vi "VoltageScan_Probecard.vi"() -> ()   [LabVIEW 2016]
uses:
  <vilib>/Utility/file.llb/Read Delimited Spreadsheet (DBL).vi
  <instrlib>/Keithley 24XX/Public/Data/Read (Single Point).vi
  <vilib>/Utility/file.llb/Write Delimited Spreadsheet (string).vi
  <instrlib>/Keithley 24XX/Keithley 24XX.lvlib
  <instrlib>/Agilent 428X Series/Agilent 428X Series.lvlib
panel:
  in  "Stop":bool
  in  "Sensor type":enum16{"6''", "8''", "One channel"}(ring)
  out "Channels":cluster{i32[], dbl[]}[](graph) caption="XY Graph"
  in  "Voltage Delay (s)":dbl=0.5 format="%#_13g"
  out "Secondary Value":dbl format="%^.4e"
  out "Primary Value":dbl format="%^.4e"
  out "Data Status":bool=TRUE
  in  "VISA resource name LCR":refnum<visa-resource-name>
  in  "Short (F:OFF)":bool
  in  "Open (F:OFF)":bool
  in  "Imp Type (0: CPD)":u32(ring) items=["CPD", "CPQ", "CPG", "CPRP", "CSD", "CSQ", "CSRS", "LPQ", "LPD", "LPG", "LPRP", "LSD", "LSQ", "LSRS", "RX", "ZTD", "ZTR", "GB", "YTD", "YTR"]
  in  "Freq Value (Hz)(1.0 kHz)":dbl=1000.0 min=20.0 max=30000000.0 step=10.0 format="%.4e"
  in  "Voltage Level (V)(1.0V)":dbl=1.0 min=0.0 max=20.0 step=0.1 format="%.4f"
  in  "Compliance  Level (uA)":dbl=0.1
  in  "Enable Voltage Auto Range (T:Enable)":bool=TRUE
  in  "Voltage Manual Range (1.0)":dbl=1.0
  in  "Serial Configuration":T1={"Baud Rate"=9600, "Parity"=0, "Data Bits"=8, "Stop Bits"=10, "Flow Control"=0} {"Flow Control" items=["None", "XON/XOFF", "RTS/CTS", "XON/XOFF & RTS/CTS", "DTR/DSR", "XON/XOFF & DTR/DSR"]; "Stop Bits" items=["1.0"=10, "1.5"=15, "2.0"=20]; "Data Bits" items=["7"=7, "8"=8]; "Parity" items=["None", "Odd", "Even", "Mark", "Space"]; "Baud Rate" items=["300"=300, "600"=600, "1200"=1200, "2400"=2400, "4800"=4800, "9600"=9600, "19200"=19200]}
  in  "VISA resource name":refnum<visa-resource-name>
  out "error out":errorcluster
  in  "Open after execution?":bool
  out "Output file":path
  in  "Output file":string="test.txt"
  out "Current voltage [V]":dbl
  out "Current channel":i32
  in  "Switch Delay (s)":dbl=0.01 format="%#_13g"
  out "Voltages":cluster{"X":dbl[], "Y":dbl[]}[](graph) caption="XY Graph"
  out "Input file":path
  in  "Measurement type":enum16{"IV", "CV", "Test"}(ring)=enum."Test"
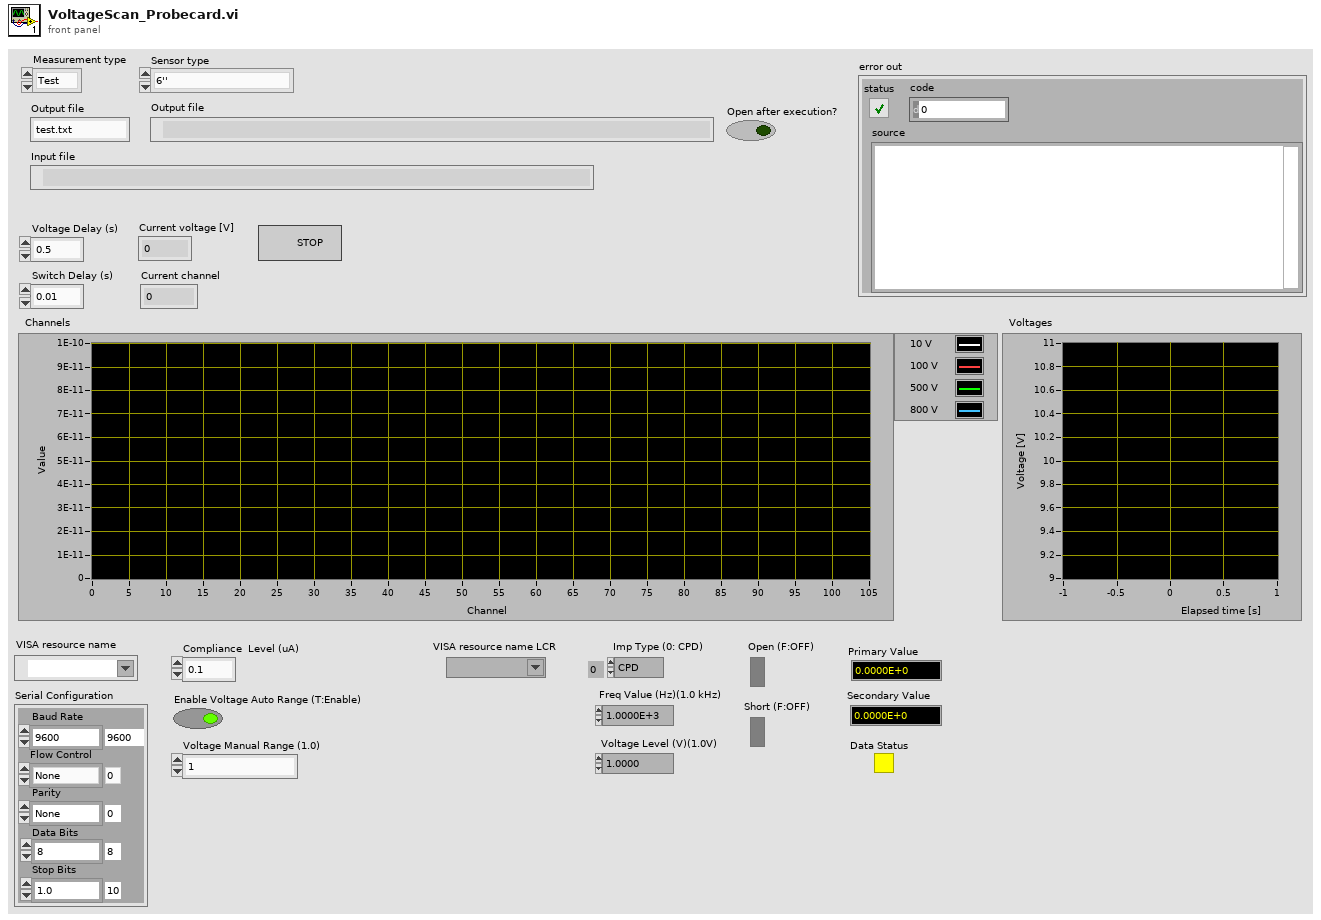
[diagram p1: front panel]
types:
  T1 = cluster{"Baud Rate":u32, "Parity":u16, "Data Bits":u16, "Stop Bits":u16, "Flow Control":u16}
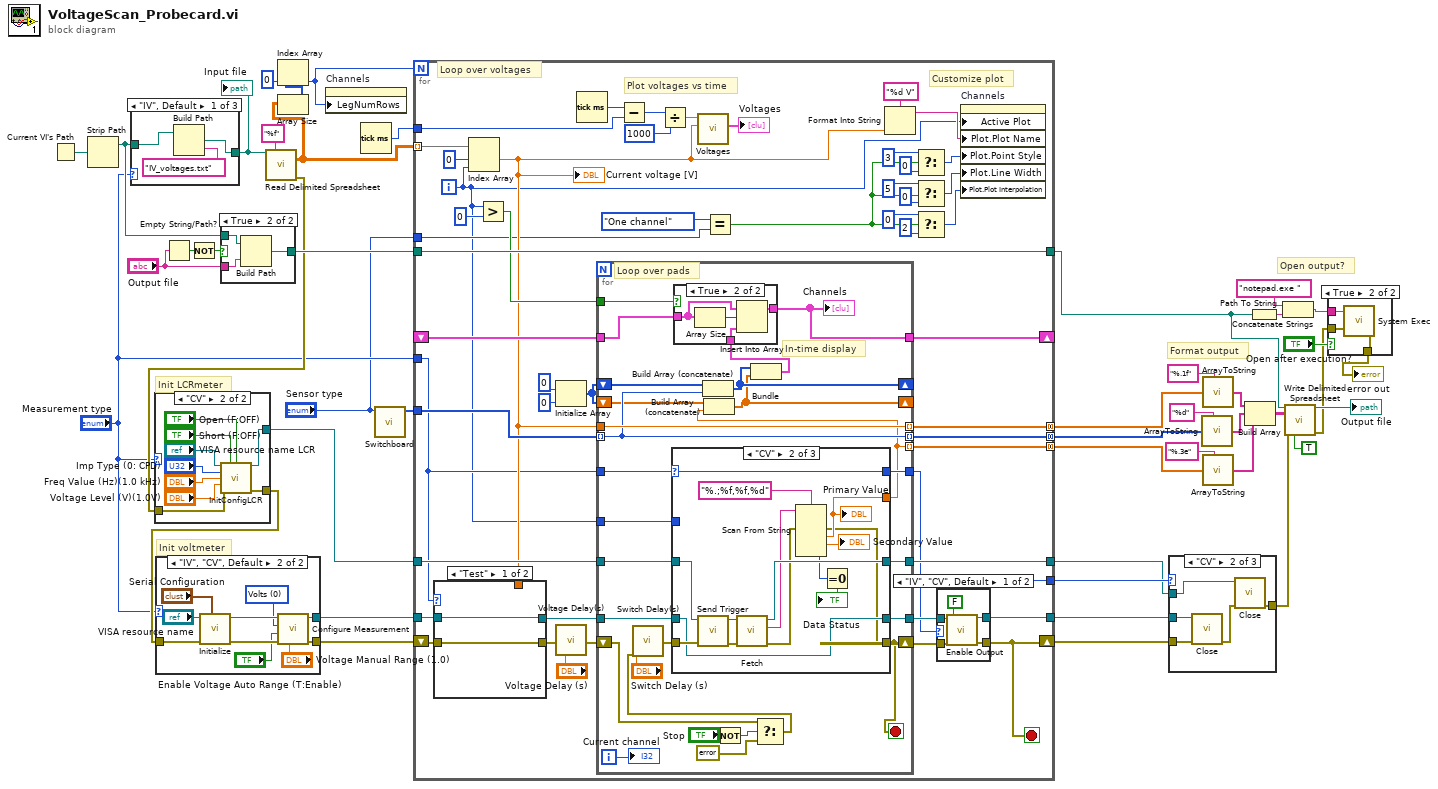
[diagram p0: block diagram]
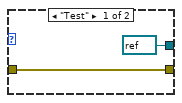
[diagram p2: hidden frame]
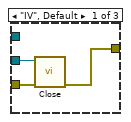
[diagram p3: hidden frame]
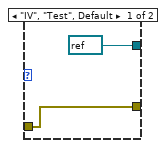
[diagram p5: hidden frame]
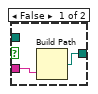
[diagram p7: hidden frame]
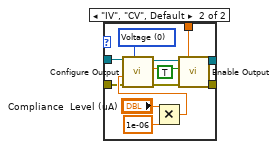
[diagram p9: hidden frame]
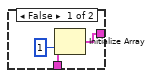
[diagram p10: hidden frame]
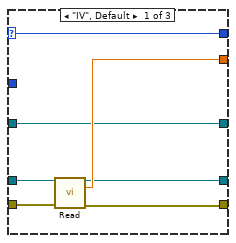
[diagram p11: hidden frame]
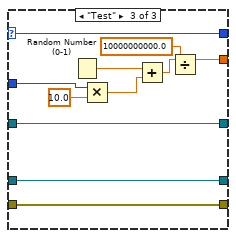
[diagram p12: hidden frame]
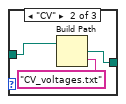
[diagram p13: hidden frame]
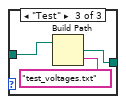
[diagram p14: hidden frame]
diagram:
  # "Init LCRmeter"
  # "Init voltmeter"
  # "Format output"
  # "Open output?"
  n1 = Current VI's Path() -> (path=w44:path)
  n2 = Strip Path(path=w44) -> (stripped path=w38:path)  [unwired: 1 out]
  n3 = case shown="\"IV\", Default" "Measurement type" {
    tunnel: [w46 w49 w52] -> w19
    tunnel: w38 -> [w48 w50 w53]
    frame "IV", Default {
      n4 = Build Path(base path=w48, name or relative path="IV_voltages.txt") -> (appended path=w46:path)
    }
    frame "CV" {
      n5 = Build Path(base path=w50, name or relative path="CV_voltages.txt") -> (appended path=w49:path)
    }
    frame "Test" {
      n6 = Build Path(base path=w53, name or relative path="test_voltages.txt") -> (appended path=w52:path)
    }
  }
  "Input file" <- w19
  n7 = Empty String/Path?(string/path="Output file") -> (empty?=w36:bool)
  n8 = Not(x=w36) -> (.not. x?=w34:bool)
  n9 = case shown="True" w34 {
    tunnel: "Output file" -> [w56 w59]
    tunnel: w38 -> [_ w58]
    tunnel: [w55 w57] -> w16
    frame False {
      n10 = Build Path(name or relative path=w56) -> (appended path=w55:path)  [unwired: 1 in]
    }
    frame True {
      n11 = Build Path(base path=w58, name or relative path=w59) -> (appended path=w57:path)
    }
  }
  n12 = call-poly <vilib>:"Read Delimited Spreadsheet.vi"("file path (dialog if empty)"=w19, "format (%.3f)"="%f") -> ("all rows"=w41:dbl[][], "error out"=w12:errorcluster)  [unwired: 8 in, 4 out]
  n13 = case shown="\"CV\"" "Measurement type" {
    tunnel: w12 -> [w61 w64]
    tunnel: [w61 w63] -> w11
    tunnel: [refnum<visa-resource-name> refnum ("VISA resource name out") w62] -> w10
    frame "IV", "Test", Default {
    }
    frame "CV" {
      n14 = call "InitConfigLCR.vi"("VISA resource name LCR"="VISA resource name LCR", "Short (F:OFF)"="Short (F:OFF)", "Open (F:OFF)"="Open (F:OFF)", "Imp Type (0: CPD)"="Imp Type (0: CPD)", "Freq Value (Hz)(1.0 kHz)"="Freq Value (Hz)(1.0 kHz)", "Voltage Level (V)(1.0V)"="Voltage Level (V)(1.0V)", "error in (no error)"=w64) -> ("VISA resource name out"=w62:refnum<visa-resource-name>, "error out"=w63:errorcluster)  [unwired: 7 in]
    }
  }
  n15 = case shown="\"IV\", \"CV\", Default" "Measurement type" {
    tunnel: [refnum<visa-resource-name> refnum ("VISA resource name out") w76] -> w15
    tunnel: [w72 w75] -> w14
    tunnel: w11 -> [w72 w74]
    frame "Test" {
    }
    frame "IV", "CV", Default {
      w79 = u16 0 items=["Volts", "Current", "Resistance"] ("Function (0: Volts)")
      n16 = call <instrlib>:"Initialize.vi"("Serial Configuration"="Serial Configuration", "error in (no error)"=w74, "VISA resource name"="VISA resource name") -> ("error out"=w80:errorcluster, "VISA resource name out"=w81:refnum<visa-resource-name>)  [unwired: 7 in]
      n17 = call <instrlib>:"Configure Measurement.vi"("Manual Range (1.0)"="Voltage Manual Range (1.0)", "error in (no error)"=w80, "Enable Auto Range (T:Enable)"="Enable Voltage Auto Range (T:Enable)", "Function (0: Volts)"=w79, "VISA resource name"=w81) -> ("error out"=w75:errorcluster, "VISA resource name out"=w76:refnum<visa-resource-name>)  [unwired: 5 in]
    }
  }
  n18 = Array Size(array=w41) -> (size(s)=w43:i32[])
  n19 = Index Array(array=w43, index=0) -> (element=w2:i32)
  n20 = property on="Channels" class="XYGraph (strict)"("LegNumRows"=w2) -> ()  [unwired: 2 in, 2 out]
  n21 = Tick Count (ms)() -> (millisecond timer value=w4:u32)
  n22 = call "Switchboard.vi"("Sensor type"="Sensor type") -> ("Output config"=w40:i32[])  [unwired: 10 in]
  n23 = for {
    N: w2 -> [_]
    tunnel: w41 -> [w132] mode=indexing
    tunnel: w40 -> [w129]
    tunnel: [w127] -> w26 mode=concatenating
    tunnel: [w125] -> w24 mode=concatenating
    tunnel: [w126] -> w25 mode=concatenating
    tunnel: w16 -> [w124]
    tunnel: [w124] -> w13
    tunnel: w15 -> [w123]
    tunnel: [w122] -> w5
    tunnel: "Measurement type" -> [w96]
    shift-right: [w100] -> w3
    shift-left: w14 -> [w117]
    tunnel: w10 -> [w116]
    tunnel: [w112] -> w9
    tunnel: [w118] -> w8
    shift-right: [w110] -> _
    shift-left: _ -> [w109]
    tunnel: w4 -> [w103]
    tunnel: "Sensor type" -> [w94]
    i -> [w83]
    stop <- w100 stop-if-true
    # "Plot voltages vs time"
    # "Customize plot"
    # "Loop over voltages"
    n24 = Index Array(array=w132, index #1=0 ("index"), index #2=w83) -> (element #1=w97:dbl)  [unwired: 1 out]
    "Current voltage [V]" <- w97
    n25 = case shown="\"Test\"" w96 {
      tunnel: w123 -> [w141 w146]
      tunnel: w97 -> [_ w145]
      tunnel: [w141 w144] -> w121
      tunnel: w117 -> [w140 w143]
      tunnel: [w140 w142] -> w114
      frame "Test" {
      }
      frame "IV", "CV", Default {
        w150 = u16 0 items=["Voltage", "Current"] ("Source Mode  (0: Voltage)")
        n26 = Multiply(x="Compliance  Level (uA)", y=1e-06) -> (x*y=w147:dbl)
        n27 = call <instrlib>:"Configure Output.vi"("Source Mode  (0: Voltage)"=w150, "error in (no error)"=w143, "Compliance  Level (0.1)"=w147, "Output Level (0)"=w145, "VISA resource name"=w146) -> ("error out"=w152:errorcluster, "VISA resource name out"=w153:refnum<visa-resource-name>)  [unwired: 5 in]
        n28 = call <instrlib>:"Enable Output.vi"("error in (no error)"=w152, "Enable Output (T: Enable)"=TRUE ("Enable Output"), "VISA resource name"=w153) -> ("error out"=w142:errorcluster, "VISA resource name out"=w144:refnum<visa-resource-name>)  [unwired: 7 in]
      }
    }
    n29 = Greater?(x=w83, y=0) -> (0:w111:bool)
    n30 = Initialize Array(0 ("dimension size"), 0 ("dimension size")) -> (w106:i32[])
    n31 = call "Voltage Delay(s)"("error in (no error)"=w114, "Delay Time (s)"="Voltage Delay (s)") -> ("error out"=w113:errorcluster)  [unwired: 9 in]
    n32 = Tick Count (ms)() -> (millisecond timer value=w105:u32)
    n33 = for {
      tunnel: w129 -> [w172] mode=indexing
      tunnel: [w172] -> w126 mode=indexing
      tunnel: [w170] -> w125 mode=indexing
      tunnel: w97 -> [w180]
      tunnel: [w180] -> w127 mode=indexing
      tunnel: w121 -> [w178]
      tunnel: [w177] -> w119
      tunnel: w96 -> [w179]
      shift-right: [w154] -> w120
      shift-left: w113 -> [w157]
      tunnel: w116 -> [w176]
      tunnel: [w175] -> w112
      tunnel: [w174] -> w118
      shift-right: [w168] -> _
      shift-left: w106 -> [w171]
      shift-right: [w167] -> _
      shift-left: w106 -> [w169]
      tunnel: w111 -> [w165]
      tunnel: w83 -> [w166]
      tunnel: w109 -> [w164]
      tunnel: [w162] -> w110
      i -> [w163]
      stop <- w154 stop-if-true
      # "In-time display"
      # "Loop over pads"
      n34 = Build Array (concatenate)(w171, w172) -> (w168:i32[])
      n35 = Not(x="Stop") -> (.not. x?=w158:bool)
      n36 = Select(t=w157, s=w158, f=errorcluster {"status"=TRUE, "code"=1, "source"="User stop"} ("User stop error")) -> (s? t:f=w155:errorcluster)
      n37 = call "Switch Delay(s)"("error in (no error)"=w155, "Delay Time (s)"="Switch Delay (s)") -> ("error out"=w156:errorcluster)  [unwired: 9 in]
      n38 = case shown="\"CV\"" w179 {
        selector: w179 -> [w189 w206 w220]
        tunnel: [w194 w198 w211] -> w170
        tunnel: w178 -> [w192 w197 w218]
        tunnel: w156 -> [w193 w204 w217]
        tunnel: [w191 w197 w218] -> w177
        tunnel: [w190 w195 w217] -> w154
        tunnel: w176 -> [w188 w207 w219]
        tunnel: [w189 w206 w220] -> w175
        tunnel: [w188 w205 w219] -> w174
        tunnel: w166 -> [_ _ w212]
        frame "IV", Default {
          n39 = call-poly <instrlib>:"Read.vi"("VISA resource name"=w192, "error in (no error)"=w193) -> ("VISA resource name out"=w191:refnum<visa-resource-name>, "Current"=w194:sgl, "error out"=w190:errorcluster)  [unwired: 7 in, 4 out]
        }
        frame "CV" {
          n40 = call <instrlib>:"Send Trigger.vi"("error in (no error)"=w204, "VISA resource name"=w207) -> ("error out"=w208:errorcluster, "VISA resource name out"=w209:refnum<visa-resource-name>)  [unwired: 8 in]
          n41 = call <instrlib>:"Fetch.vi"("error in (no error)"=w208, "VISA resource name"=w209) -> ("error out"=w196:errorcluster, "Returned Data"=w199:string, "VISA resource name out"=w205:refnum<visa-resource-name>)  [unwired: 7 in]
          n42 = Scan From String(format string="%.;%f,%f,%d", input string=w199, error in=w196) -> (error out=w195:errorcluster, output 1=w198:dbl, output 2=→"Secondary Value":dbl, output 3=w203:i32)  [unwired: 4 in, 2 out]
          "Primary Value" <- w198
          n43 = Equal To 0?(x=w203) -> (x = 0?=→"Data Status":bool)
        }
        frame "Test" {
          n44 = Random Number (0-1)() -> (number: 0 to 1=w216:dbl)
          n45 = Multiply(x=w212, y=10.0) -> (x*y=w213:dbl)
          n46 = Add(x=w216, y=w213) -> (x+y=w215:dbl)
          n47 = Divide(x=w215, y=10000000000.0) -> (x/y=w211:dbl)
        }
      }
      n48 = Build Array (concatenate)(w169, w170) -> (w167:dbl[])
      n49 = Bundle(w168, w167) -> (w161:cluster{i32[], dbl[]})  [unwired: 1 out]
      n50 = case shown="True" w165 {
        tunnel: w164 -> [_ w186]
        tunnel: [w181 w185] -> w162
        tunnel: w161 -> [w182 w184]
        frame False {
          n51 = Initialize Array(w182, 1 ("dimension size")) -> (w181:cluster{i32[], dbl[]}[])
        }
        frame True {
          n52 = Array Size(array=w186) -> (size(s)=w187:i32)
          n53 = Insert Into Array(array=w186, index=w187, new element=w184) -> (w185:cluster{i32[], dbl[]}[])
        }
      }
      "Channels" <- w162
      "Current channel" <- w163
    }
    n54 = Subtract(x=w105, y=w103) -> (x-y=w104:u32)
    n55 = Divide(x=w104, y=u32 1000 ("x")) -> (x/y=w102:dbl)
    n56 = call "Voltages"("Y Input"=w97, "X Input"=w102) -> ("XY Graph"=→"Voltages":cluster{"X":dbl[], "Y":dbl[]}[])  [unwired: 8 in, 1 out]
    n57 = Equal?(x=enum16{"6''", "8''", "One channel"}."One channel" ("Sensor type 2"), y=w94) -> (x = y?=w85:bool)
    n58 = Format Into String(format string="%d V", w97) -> (resulting string=w99:string)  [unwired: 2 in, 1 out]
    n59 = Select(t=u8 3 ("Plot.Point Style"), s=w85, f=u8 0 ("Plot.Point Style")) -> (s? t:f=w90:u8)
    n60 = Select(t=u8 5 ("Plot.Point Style"), s=w85, f=u8 0 ("Plot.Point Style")) -> (s? t:f=w88:u8)
    n61 = Select(t=u8 0 ("Plot.Point Style"), s=w85, f=u8 2 ("Plot.Point Style")) -> (s? t:f=w84:u8)
    n62 = case shown="\"IV\", \"CV\", Default" w112 {
      tunnel: [w136 w139] -> w122
      tunnel: w120 -> [w135 w138]
      tunnel: w119 -> [w134 w139]
      tunnel: [w133 w138] -> w100
      frame "IV", "CV", Default {
        n63 = call <instrlib>:"Enable Output.vi"("error in (no error)"=w135, "Enable Output (T: Enable)"=FALSE ("Enable Output"), "VISA resource name"=w134) -> ("error out"=w133:errorcluster, "VISA resource name out"=w136:refnum<visa-resource-name>)  [unwired: 7 in]
      }
      frame "Test" {
      }
    }
    n64 = property on="Channels" class="XYGraph (strict)"("Active Plot"=w83, "Plot.Plot Name"=w99, "Plot.Point Style"=w90, "Plot.Line Width"=w88, "Plot.Plot Interpolation"=w84) -> ()  [unwired: 2 in, 2 out]
  }
  n65 = case shown="\"CV\"" w9 {
    tunnel: w8 -> [_ w228 _]
    tunnel: w3 -> [w222 w226 w229]
    tunnel: [w221 w227 w229] -> w7
    tunnel: w5 -> [w223 w224 _]
    frame "IV", Default {
      n66 = call <instrlib>:"Close.vi"("error in (no error)"=w222, "VISA resource name"=w223) -> ("error out"=w221:errorcluster)  [unwired: 9 in]
    }
    frame "CV" {
      n67 = call <instrlib>:"Close.vi"("error in (no error)"=w226, "VISA resource name"=w224) -> ("error out"=w225:errorcluster)  [unwired: 9 in]
      n68 = call <instrlib>:"Close.vi"("error in (no error)"=w225, "VISA resource name"=w228) -> ("error out"=w227:errorcluster)  [unwired: 9 in]
    }
    frame "Test" {
    }
  }
  n69 = call "ArrayToString.vi"("Format"="%d", "Input 1D array"=w25) -> ("Output 1D array"=w28:string[])  [unwired: 7 in]
  n70 = call "ArrayToString.vi"("Format"="%.1f", "Input 1D array"=w26) -> ("Output 1D array"=w29:string[])  [unwired: 7 in]
  n71 = call "ArrayToString.vi"("Format"="%.3e", "Input 1D array"=w24) -> ("Output 1D array"=w30:string[])  [unwired: 7 in]
  n72 = Build Array(w29, w28, w30) -> (w27:string[][])
  n73 = Path To String(path=w13) -> (string=w23:string)
  n74 = Concatenate Strings("notepad.exe " ("string"), w23) -> (w21:string)
  n75 = call-poly <vilib>:"Write Delimited Spreadsheet.vi"("file path (dialog if empty)"=w13, "2D data"=w27, "error in (no error)"=w7, "transpose? (no:F)"=TRUE) -> ("new file path (Not A Path if cancelled)"=→"Output file":path, "error out"=w18:errorcluster)  [unwired: 10 in]
  n76 = case shown="True" "Open after execution?" {
    tunnel: w21 -> [_ w233]
    tunnel: w18 -> [w230 w232]
    tunnel: [w230 w231] -> w17
    frame False {
    }
    frame True {
      n77 = call <vilib>:"System Exec.vi"("error in (no error)"=w232, "command line"=w233) -> ("error out"=w231:errorcluster)  [unwired: 6 in, 3 out]
    }
  }
  "error out" <- w17
